vi "Save to File_input_filename.vi"(1 "data":waveform(dbl)[](array[waveform]), 2 "Save to File":bool) -> (0 "File Name Out Location":path caption="File Name Out")   [LabVIEW 2013]
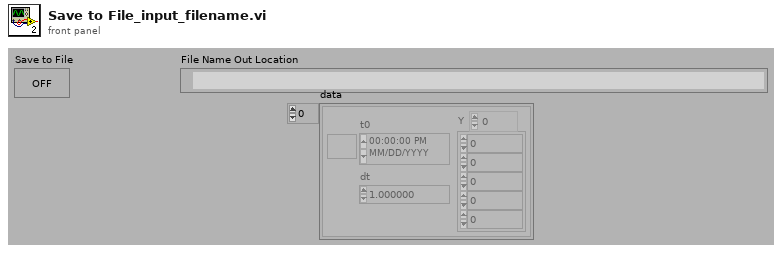
[diagram p1: front panel]
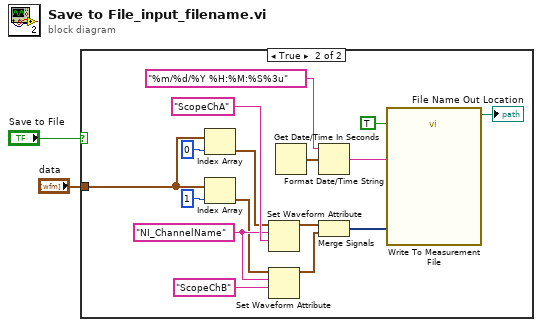
[diagram p0: block diagram]
diagram:
  n1 = case shown="True" "Save to File" {
    tunnel: "data" -> [_ w7]
    frame False {
    }
    frame True {
      w14 = "NI_ChannelName"
      n2 = Index Array(array=w7, index=0 ("index (row)")) -> (element=w6:waveform(dbl))
      n3 = Index Array(array=w7, index=1 ("index (row)")) -> (element=w5:waveform(dbl))
      n4 = Set Waveform Attribute(5:"ScopeChA", 6:w14, 7:w6) -> (3:w13:waveform(dbl))  [unwired: 1 in, 2 out]
      n5 = Set Waveform Attribute(5:"ScopeChB", 6:w14, 7:w5) -> (3:w12:waveform(dbl))  [unwired: 1 in, 2 out]
      n6 = Get Date/Time In Seconds() -> (seconds since 1Jan1904=w10:timestamp)
      n7 = Format Date/Time String(time format string (%c)="%m/%d/%Y %H:%M:%S%3u", seconds (now)=w10) -> (date/time string=w8:string)  [unwired: 1 out]
      n8 = Merge Signals(w13, w12) -> (w11:dynamicdata)
      n9 = call "Write To Measurement File"("Signals"=w11, "Reset"=TRUE, "Comment"=w8) -> ("Filename Out"=→"File Name Out Location":path)  [unwired: 14 in, 2 out]
    }
  }
